vi "AlliGator Load Phasor Plots v3.vi"(8 "Error In":errorcluster, 10 "File paths":path[](array[path]) caption="selected paths", 11 "XYGraph in":refnum<vi>) -> (0 "Error Out":errorcluster, 1 "Last Raw Phasor Plot":cluster{"g":dbl[], "s":dbl[]}, 2 "Message":string, 3 "Raw Phasor Plot":T1[](array[typedef]) {"[Decay Metadata]"."# Folds" min=1; "[Decay Metadata]"."ROI Descriptor"."Contours"."Type" items=["No Selection", "Point", "Line", "Rectangle", "Oval", "Polygon", "Freehand Region", "Annulus", "Unused2", "Unused3", "Broken Line", "Freehand Line", "Rotated Rectangle"]})   [LabVIEW 2021, in "AlliGator Phasor Graph.lvlib"]
doc: "Loads Phasor Plot(s) and associated data and metadata from a phplot file.\n\nIf no file paths are provided, a dialog window is shown."
uses:
  AlliGator Phasor Graph.lvlib
  AlliGator Raw Phasor Plot Data v4.ctl
  Phasor/Phasor (g, s).ctl
  AlliGator Decay Metadata v3.ctl
  AlliGator Decay Background Subtraction Info.ctl
  AlliGator Baseline Subtraction Method.ctl
  Graphs/XY Graph/XY Graph Plot Shift Parameters.ctl
  Graphs/XY Graph/XY Graph Plot Shift Method.ctl
  AlliGator Decay Extrapolation Parameters.ctl
  Phasor/Phasor Standard Deviation Options.ctl
  Phasor/Calibration Phasor (m, phi).ctl
  Graphs/LabVIEW Plot Interpolation.ctl
  Graphs/Plot Point Style.ctl
  AlliGator Raw Phasor Plot Data v2.ctl
  AlliGator Decay Metadata.ctl
  AlliGator Raw Phasor Plot Data v1.ctl
  AlliGator Raw Phasor Plot Data v3.ctl
  068f6334-c7bc-4b58-b106-ea81d4237ab9.vi
  4623fcf5-0913-4af6-b274-a61fc63dc5a4.vi
  d75a8ec3-395c-45c9-858a-6d0515c4ea0f.vi
  9735f987-b6b5-414e-80a6-54cad8db5d94.vi
  <vilib>/Utility/error.llb/Error Cluster From Error Code.vi
  <vilib>/JDP Science/JSONtext/JSON text to Variant.vi
  Utilities/Logical Processors Used.vi
  Graphs/XY Graph/XY Graph Add Single Plot with Name.vi
  <vilib>/ErrorRing/Error Ring.xnode
  <vilib>/JDP Science/JSONtext/LVClass Serializer/JSONtext LVClass Serializer.lvclass
  Graphs/XY Graph/XY Graph Add-Ons.lvlib
  Phasor/Phasor.lvlib
  Files/Files.lvlib
  Graphs/Graphs.lvlib
  AlliGator Decay Preprocessing.lvlib
  Strings/Strings.lvlib
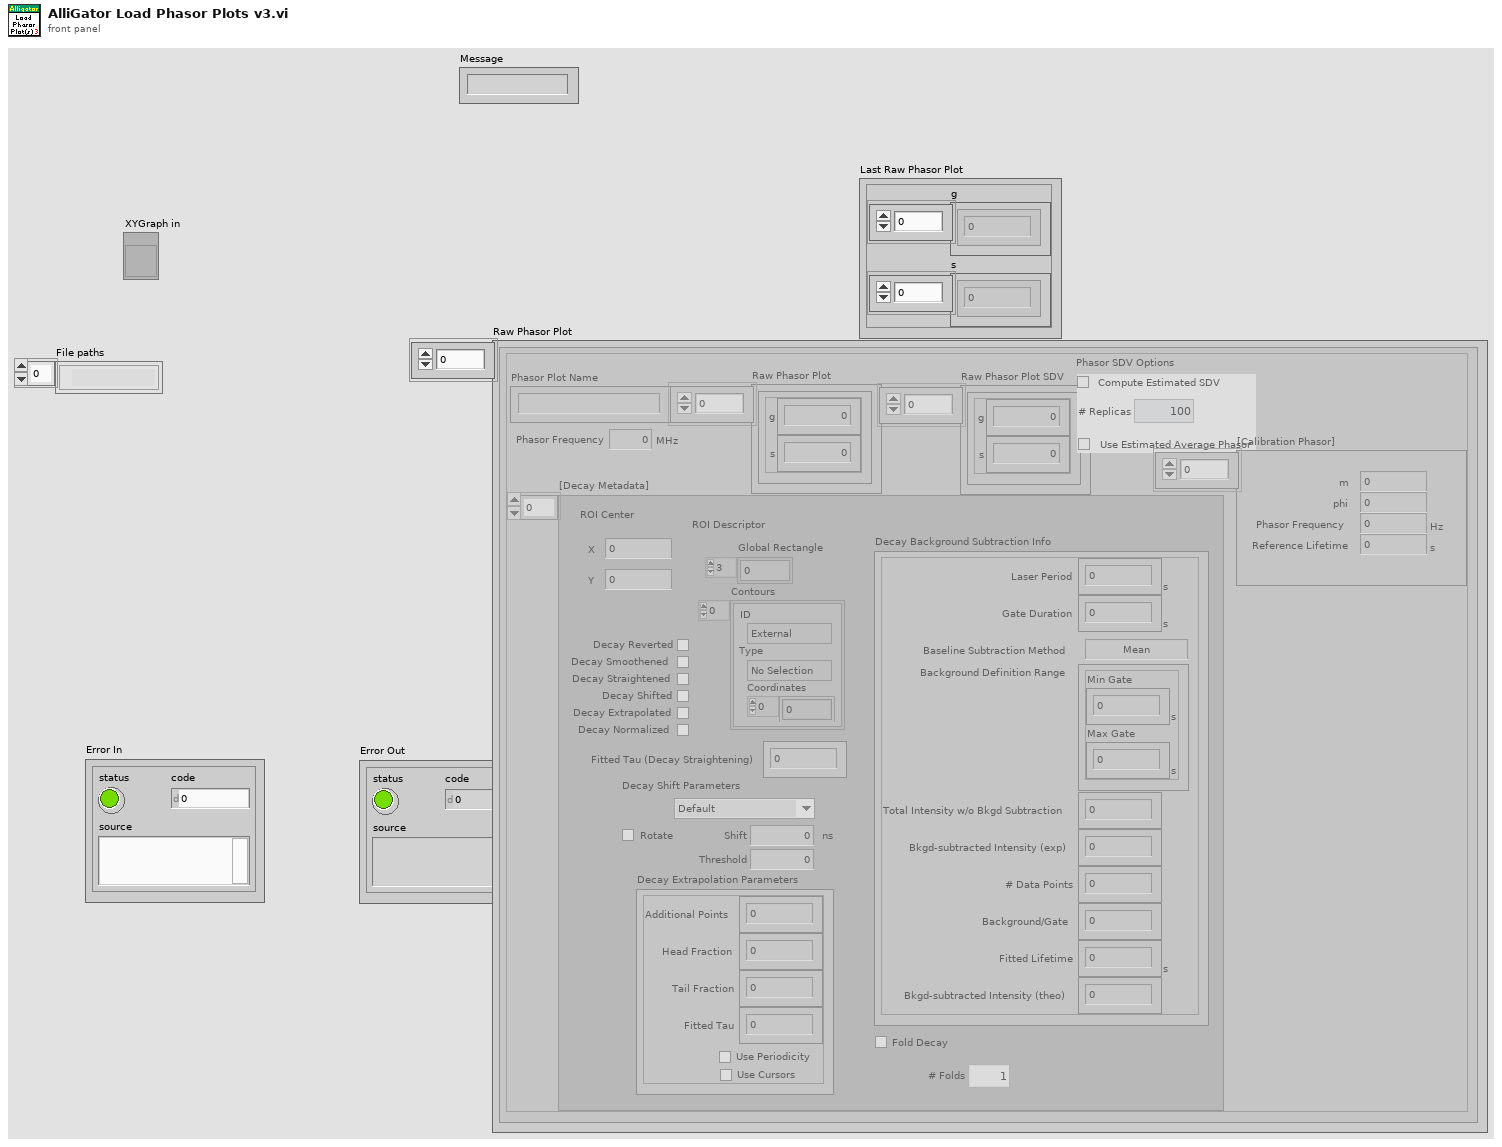
[diagram p1: front panel]
types:
  T1 = typedef "AlliGator Phasor Graph.lvlib/AlliGator Raw Phasor Plot Data v4.ctl" = cluster{"Phasor Plot Name":string, "Raw Phasor Plot":T2[], "Phasor Frequency":dbl[unit], "[Decay Metadata]":T3[], "Raw Phasor Plot SDV":T2[], "Phasor SDV Options":T10, "[Calibration Phasor]":T11[]}
  T2 = typedef "Phasor.lvlib/Phasor (g, s).ctl" = cluster{"g":dbl, "s":dbl}
  T3 = typedef "AlliGator Phasor Graph.lvlib/AlliGator Decay Metadata v3.ctl" = cluster{"ROI Descriptor":T4, "ROI Center":cluster{"X":i32, "Y":i32}, "Decay Background Subtraction Info":T5, "Decay Reverted":bool, "Decay Smoothened":bool, "Decay Straightened":bool, "Fitted Tau (Decay Straightening)":dbl, "Decay Shift Parameters":T7, "Decay Shifted":bool, "Decay Extrapolated":bool, "Decay Extrapolation Parameters":T9, "Decay Normalized":bool, "Fold Decay":bool, "# Folds":u32}
  T4 = typedef "ROI Descriptor" = cluster{"Global Rectangle":i32[], "Contours":cluster{"ID":enum32{"External", "Internal"}, "Type":u32, "Coordinates":i32[]}[]}
  T5 = typedef "AlliGator Decay Analysis.lvlib/AlliGator Decay Preprocessing.lvlib/AlliGator Decay Background Subtraction Info.ctl" = cluster{"Laser Period":dbl[unit], "Gate Duration":dbl[unit], "Baseline Subtraction Method":T6, "Background Definition Range":cluster{"Min Gate":dbl[unit], "Max Gate":dbl[unit]}, "Total Intensity w/o Bkgd Subtraction":dbl, "Bkgd-subtracted Intensity (exp)":dbl, "# Data Points":i32, "Background/Gate":dbl, "Fitted Lifetime":dbl[unit], "Bkgd-subtracted Intensity (theo)":dbl}
  T6 = typedef "AlliGator Decay Analysis.lvlib/AlliGator Decay Preprocessing.lvlib/AlliGator Baseline Subtraction Method.ctl" = enum16{"Mean", "Min", "Square Gated Single-Exponential", "File", "Constant"}
  T7 = typedef "XY Graph Add-Ons.lvlib/XY Graph Plot Shift Parameters.ctl" = cluster{"Type":T8, "Shift":dbl[unit], "Threshold":dbl, "Rotate":bool}
  T8 = typedef "XY Graph Add-Ons.lvlib/XY Graph Plot Shift Method.ctl" = enum16{"Default", "CFD", "Threshold", "Cross-Correlation"}
  T9 = typedef "AlliGator Decay Analysis.lvlib/AlliGator Decay Preprocessing.lvlib/AlliGator Decay Extrapolation Parameters.ctl" = cluster{"Additional Points":u32, "Head Fraction":dbl, "Fitted Tau":dbl, "Use Periodicity":bool, "Use Cursors":bool, "Tail Fraction":dbl}
  T10 = typedef "Phasor.lvlib/Phasor Standard Deviation Options.ctl" = cluster{"Compute Estimated SDV":bool, "# Replicas":u32, "Use Estimated Average Phasor":bool}
  T11 = typedef "Phasor.lvlib/Calibration Phasor (m, phi).ctl" = cluster{"m":dbl, "phi":dbl, "Phasor Frequency":dbl[unit], "Reference Lifetime":dbl[unit]}
  T12 = typedef "Graphs.lvlib/Plot Point Style.ctl" = enum16{"not defined", "None", "Empty Circle", "Filled Circle", "Thick Circle", "Dotted Circle", "Empty Square", "Filled Square", "Thick Square", "Dotted Square", "Small Filled Square", "Dot", "Cross", "Tiny Cross", "Large X", "Small x", "Diamond", "Small Empty Square"}
  T13 = typedef "AlliGator Phasor Graph.lvlib/AlliGator Raw Phasor Plot Data v1.ctl" = cluster{"Plot Name":string, "Raw Phasor Plot":T2[], "Phasor Frequency":dbl[unit]}
  T14 = typedef "AlliGator Phasor Graph.lvlib/AlliGator Raw Phasor Plot Data v2.ctl" = cluster{"Plot Name":string, "Raw Phasor Plot":T2[], "Phasor Frequency":dbl[unit], "Phasor Metadata":T15[]}
  T15 = typedef "AlliGator Phasor Graph.lvlib/AlliGator Decay Metadata.ctl" = cluster{"Total Intensity":dbl, "# Gates":i32, "Background":dbl, "Amplitude":dbl, "Lifetime":dbl[unit], "Bkgd-subtracted Intensity (exp)":dbl, "Bkgd-subtracted Intensity (theo)":dbl}
  T16 = typedef "Graphs.lvlib/LabVIEW Plot Interpolation.ctl" = u8
  T17 = typedef "AlliGator Phasor Graph.lvlib/AlliGator Raw Phasor Plot Data v3.ctl" = cluster{"Plot Name":string, "Raw Phasor Plot":T2[], "Phasor Frequency":dbl[unit], "Phasor Metadata":T3[]}
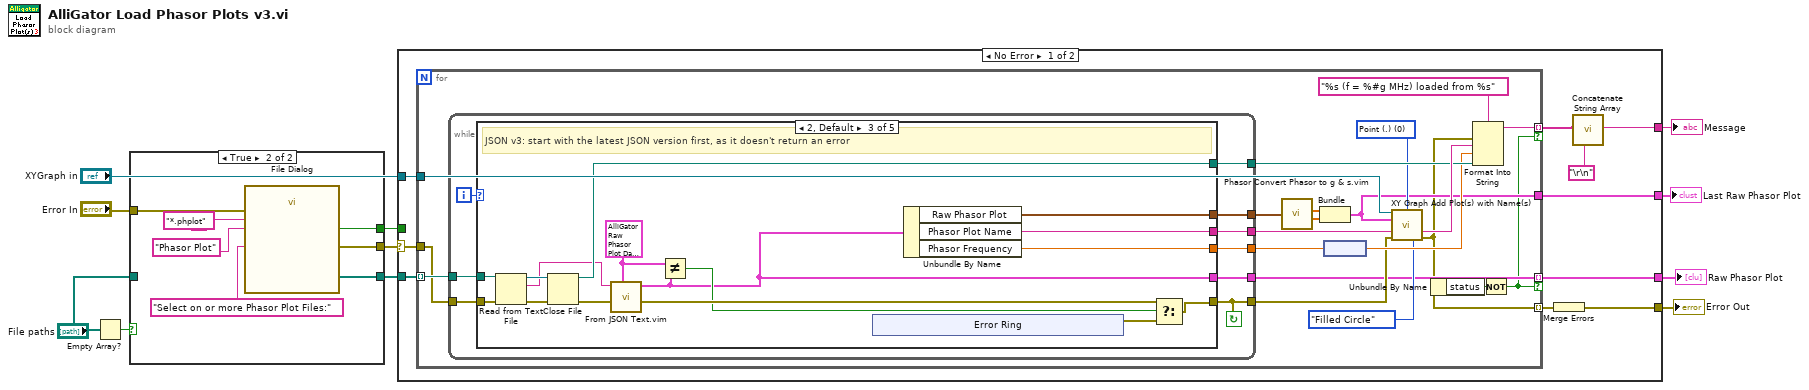
[diagram p0: block diagram]
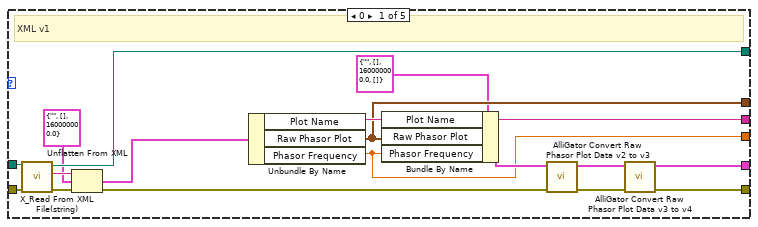
[diagram p3: hidden frame]
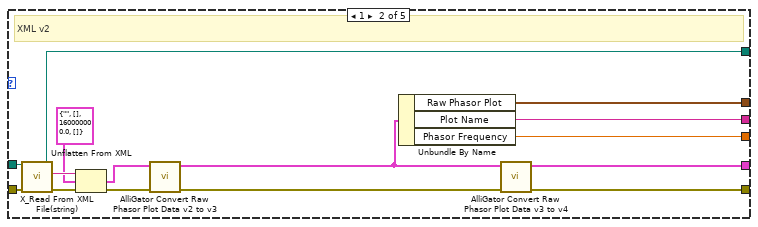
[diagram p4: hidden frame]
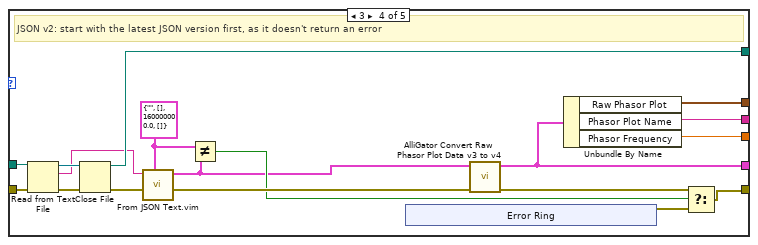
[diagram p5: hidden frame]
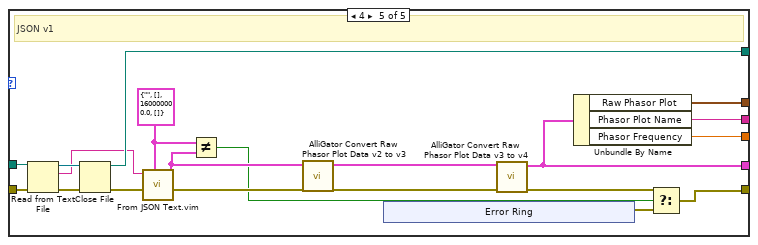
[diagram p6: hidden frame]
diagram:
  n1 = Empty Array?(array="File paths") -> (empty?=w3:bool)
  n2 = case shown="True" w3 {
    tunnel: [w13 w20] -> w9
    tunnel: [w12 w19] -> w8
    tunnel: [_ w18] -> w7
    tunnel: "Error In" -> [w12 w17]
    tunnel: "File paths" -> [w13 _]
    frame False {
    }
    frame True {
      n3 = call "File Dialog"("prompt"="Select on or more Phasor Plot Files:", "error in"=w17, "pattern (all files)"="*.phplot" ("pattern (*.phplot)"), "pattern label"="Phasor Plot") -> ("selected paths"=w20:path[], "cancelled"=w18:bool, "error out"=w19:errorcluster)  [unwired: 8 in, 1 out]
    }
  }
  n4 = case shown="No Error" w8 {
    selector: w8 -> [w26 _]
    tunnel: "XYGraph in" -> [w30 _]
    tunnel: [w28 _] -> w10
    tunnel: w9 -> [w27 _]
    tunnel: [w25 _] -> w5
    tunnel: [w24 _] -> w4
    tunnel: w7 -> [_ _]
    tunnel: [w21 _] -> w1
    frame No Error {
      n5 = for {
        tunnel: w27 -> [w50] mode=indexing
        tunnel: w30 -> [w51]
        tunnel: [w33] -> w29 mode=indexing
        tunnel: w26 -> [w49]
        tunnel: [w34] -> w25 mode=indexing if=w31
        tunnel: [w36] -> w24
        tunnel: [w32] -> w23 mode=indexing if=w31
        w38 = T16 0 items=["Point (.)", "Stepwise Right (--.)", "Line + Point (\\. /)", "Stepwise Left (.--)", "Stepwise Centered (-.-)", "Stepwise Vertical (|.|)", "Line (-)", "Use Previous Plot's Style"] ("Plot Interpolation (Previous Plot's Style)")
        n6 = while {
          tunnel: [w58] -> w48
          tunnel: [w57] -> w47
          tunnel: [w55] -> w41
          tunnel: [w54] -> w34
          tunnel: w50 -> [w60]
          tunnel: [w56] -> w42
          tunnel: w49 -> [w59]
          tunnel: [w53] -> w35
          i -> [w52]
          stop <- w53 continue-if-true
          n7 = case shown="2, Default" w52 {
            tunnel: w60 -> [w77 w92 w107 w129 w149]
            tunnel: w59 -> [w76 w91 w108 w130 w150]
            tunnel: [w75 w90 w94 w115 w153] -> w58
            tunnel: [w74 w89 w95 w116 w152] -> w57
            tunnel: [w73 w88 w104 w126 w146] -> w56
            tunnel: [w61 w87 w93 w114 w151] -> w55
            tunnel: [w62 w79 w96 w113 w135] -> w54
            tunnel: [w63 w80 w100 w122 w136] -> w53
            frame 0 {
              # "XML v1"
              n8 = call "X_Read From XML File(string).vi"("error in (no error)"=w76, "XML File Path"=w77) -> ("error out"=w71:errorcluster, "XML Elements"=w72:string, "XML File Path(duplicate)"=w73:path)  [unwired: 7 in]
              n9 = Unflatten From XML(xml string=w72, type=T13 {"Plot Name"="", "Raw Phasor Plot"=[], "Phasor Frequency"=160000000.0} ("Raw Phasor Plot Data"), error in (no error)=w71) -> (value=w68:T13, error out=w65:errorcluster)
              n10 = Unbundle By Name(w68) -> ("Plot Name"=w75:string, "Raw Phasor Plot"=w74:T2[], "Phasor Frequency"=w61:dbl[unit])
              n11 = Bundle By Name(cluster=T14 {"Plot Name"="", "Raw Phasor Plot"=[], "Phasor Frequency"=160000000.0, "Phasor Metadata"=[]} ("Raw Phasor Plot Data"), "Plot Name"=w75, "Raw Phasor Plot"=w74, "Phasor Frequency"=w61) -> (w64:T14)
              n12 = call "AlliGator Convert Raw Phasor Plot Data v2 to v3.vi"("Error In"=w65, "Raw Phasor Plot Data v2"=w64) -> ("Error Out"=w66:errorcluster, "Raw Phasor Plot Data v3"=w67:T17)  [unwired: 8 in]
              n13 = call "AlliGator Convert Raw Phasor Plot Data v3 to v4.vi"("error in (no error)"=w66, "Raw Phasor Plot Data v3"=w67) -> ("error out"=w63:errorcluster, "Raw Phasor Plot Data v4"=w62:T1)  [unwired: 8 in]
            }
            frame 1 {
              # "XML v2"
              n14 = call "X_Read From XML File(string).vi"("error in (no error)"=w91, "XML File Path"=w92) -> ("error out"=w85:errorcluster, "XML Elements"=w86:string, "XML File Path(duplicate)"=w88:path)  [unwired: 7 in]
              n15 = Unflatten From XML(xml string=w86, type=T14 {"Plot Name"="", "Raw Phasor Plot"=[], "Phasor Frequency"=160000000.0, "Phasor Metadata"=[]} ("Raw Phasor Plot Data"), error in (no error)=w85) -> (value=w83:T14, error out=w82:errorcluster)
              n16 = call "AlliGator Convert Raw Phasor Plot Data v2 to v3.vi"("Error In"=w82, "Raw Phasor Plot Data v2"=w83) -> ("Error Out"=w81:errorcluster, "Raw Phasor Plot Data v3"=w78:T17)  [unwired: 8 in]
              n17 = Unbundle By Name(w78) -> ("Raw Phasor Plot"=w89:T2[], "Plot Name"=w90:string, "Phasor Frequency"=w87:dbl[unit])
              n18 = call "AlliGator Convert Raw Phasor Plot Data v3 to v4.vi"("error in (no error)"=w81, "Raw Phasor Plot Data v3"=w78) -> ("error out"=w80:errorcluster, "Raw Phasor Plot Data v4"=w79:T1)  [unwired: 8 in]
            }
            frame 2, Default {
              w98 = T1 {"Phasor Plot Name"="", "Raw Phasor Plot"=[], "Phasor Frequency"=160000000.0, "[Decay Metadata]"=[], "Raw Phasor Plot SDV"=[], "Phasor SDV Options"={"Compute Estimated SDV"=FALSE, "# Replicas"=100, "Use Estimated Average Phasor"=FALSE}, "[Calibration Phasor]"=[]} ("Raw Phasor Plot Data")
              # "JSON v3: start with the latest JSON version first, as it doesn't return an error"
              n19 = Read from Text File(file (use dialog)=w107, error in=w108) -> (refnum out=w106:refnum<file>, text=w103:string, error out=w105:errorcluster)  [unwired: 2 in, 1 out]
              n20 = Close File(refnum=w106, error in=w105) -> (path=w104:path, error out=w102:errorcluster)
              n21 = call "From JSON Text.vim"("Data Type and Default Value"=w98, "error in (no error)"=w102, "JSON"=w103) -> ("error out"=w101:errorcluster, "Data out"=w96:T1)  [unwired: 7 in]
              n22 = Not Equal?(x=w98, y=w96) -> (x != y?=w97:bool)
              n23 = xnode "Error Ring"() -> ("error out"=w99:errorcluster)
              n24 = Unbundle By Name(w96) -> ("Raw Phasor Plot"=w95:T2[], "Phasor Plot Name"=w94:string, "Phasor Frequency"=w93:dbl[unit])
              n25 = Select(t=w101, s=w97, f=w99) -> (s? t:f=w100:errorcluster)
            }
            frame 3 {
              w119 = T17 {"Plot Name"="", "Raw Phasor Plot"=[], "Phasor Frequency"=160000000.0, "Phasor Metadata"=[]} ("Raw Phasor Plot Data")
              # "JSON v2: start with the latest JSON version first, as it doesn't return an error"
              n26 = Read from Text File(file (use dialog)=w129, error in=w130) -> (refnum out=w128:refnum<file>, text=w125:string, error out=w127:errorcluster)  [unwired: 2 in, 1 out]
              n27 = Close File(refnum=w128, error in=w127) -> (path=w126:path, error out=w124:errorcluster)
              n28 = call "From JSON Text.vim"("Data Type and Default Value"=w119, "error in (no error)"=w124, "JSON"=w125) -> ("error out"=w123:errorcluster, "Data out"=w117:T17)  [unwired: 7 in]
              n29 = Not Equal?(x=w119, y=w117) -> (x != y?=w118:bool)
              n30 = xnode "Error Ring"() -> ("error out"=w121:errorcluster)
              n31 = call "AlliGator Convert Raw Phasor Plot Data v3 to v4.vi"("error in (no error)"=w123, "Raw Phasor Plot Data v3"=w117) -> ("error out"=w120:errorcluster, "Raw Phasor Plot Data v4"=w113:T1)  [unwired: 8 in]
              n32 = Unbundle By Name(w113) -> ("Raw Phasor Plot"=w116:T2[], "Phasor Plot Name"=w115:string, "Phasor Frequency"=w114:dbl[unit])
              n33 = Select(t=w120, s=w118, f=w121) -> (s? t:f=w122:errorcluster)
            }
            frame 4 {
              w141 = T14 {"Plot Name"="", "Raw Phasor Plot"=[], "Phasor Frequency"=160000000.0, "Phasor Metadata"=[]} ("Raw Phasor Plot Data")
              # "JSON v1"
              n34 = Read from Text File(file (use dialog)=w149, error in=w150) -> (refnum out=w148:refnum<file>, text=w145:string, error out=w147:errorcluster)  [unwired: 2 in, 1 out]
              n35 = Close File(refnum=w148, error in=w147) -> (path=w146:path, error out=w144:errorcluster)
              n36 = call "From JSON Text.vim"("Data Type and Default Value"=w141, "error in (no error)"=w144, "JSON"=w145) -> ("error out"=w143:errorcluster, "Data out"=w140:T14)  [unwired: 7 in]
              n37 = Not Equal?(x=w141, y=w140) -> (x != y?=w137:bool)
              n38 = call "AlliGator Convert Raw Phasor Plot Data v2 to v3.vi"("Raw Phasor Plot Data v2"=w140) -> ("Raw Phasor Plot Data v3"=w142:T17)  [unwired: 9 in, 1 out]
              n39 = xnode "Error Ring"() -> ("error out"=w138:errorcluster)
              n40 = call "AlliGator Convert Raw Phasor Plot Data v3 to v4.vi"("error in (no error)"=w143, "Raw Phasor Plot Data v3"=w142) -> ("error out"=w139:errorcluster, "Raw Phasor Plot Data v4"=w135:T1)  [unwired: 8 in]
              n41 = Unbundle By Name(w135) -> ("Raw Phasor Plot"=w152:T2[], "Phasor Plot Name"=w153:string, "Phasor Frequency"=w151:dbl[unit])
              n42 = Select(t=w139, s=w137, f=w138) -> (s? t:f=w136:errorcluster)
            }
          }
        }
        n43 = call "Phasor Convert Phasor to g & s.vim"("Phasor Array"=w47) -> ("g"=w46:dbl[], "s"=w45:dbl[])  [unwired: 8 in]
        n44 = Bundle("g"=w46, "s"=w45) -> (w36:cluster{"g":dbl[], "s":dbl[]})  [unwired: 1 in]
        n45 = node(w41) -> (w40:dbl)
        n46 = call-poly "XY Graph Add Plot(s) with Name(s).vi"("XYGraph Ref in"=w51, "Plot Interpolation (Previous Plot's Style)"=w38, "Plot"=w36, "Plot Name (\"Plot\")"=w48, "error in (no error)"=w35, "Point Style (Dot)"=Plot_Point_Style."Filled Circle") -> ("Plot Name"=w43:string, "error out"=w33:errorcluster)  [unwired: 6 in, 2 out]
        n47 = Unbundle By Name(w33) -> ("status"=w39:bool)
        n48 = Format Into String(format string="%s (f = %#g MHz) loaded from %s", error in=w33, w43, w40, w42) -> (resulting string=w32:string)  [unwired: 1 in, 1 out]
        n49 = Not(x=w39) -> (.not. x?=w31:bool)
      }
      n50 = Merge Errors(w29) -> (w28:errorcluster)
      n51 = call "Concatenate String Array.vi"("Separator (TAB)"="\r\n", "String Array"=w23) -> ("Formatted String"=w21:string)  [unwired: 9 in]
    }
    frame Error {
    }
  }
  "Error Out" <- w10
  "Raw Phasor Plot" <- w5
  "Last Raw Phasor Plot" <- w4
  "Message" <- w1
